vi "Read extParam.vi"(8 "error in":errorcluster, 11 "CRDS Cell Data in":refnum<class "CRDS Cell Data.lvclass">) -> (0 "error out":errorcluster, 2 "extParam":T1={"Tau"=nan, "Tau0cor"=nan, "ext"=nan, "extCorr"=nan, "stdevTau"=nan, "eTau"=nan, "taucorr"=nan, "Tau0"=nan, "max"=nan}, 3 "CRDS Cell Data out":refnum<class "CRDS Cell Data.lvclass">)   [LabVIEW 2018, in "CRDS Lib.lvlib" / "CRDS Cell Data.lvclass"]
uses:
  CRDS Cell Data.lvclass
  Cell/extParam Ctl.ctl
  CRDS Cell Data.lvclass/CRDS Cell Data.ctl
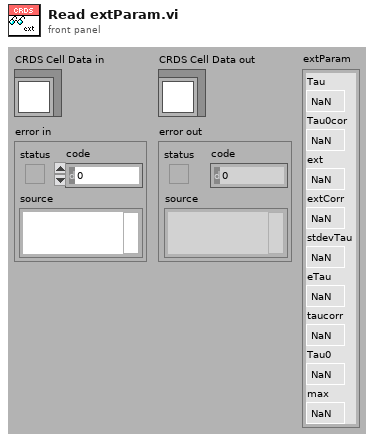
[diagram p1: front panel]
types:
  T1 = typedef "CRDS Lib.lvlib/CRDS Cell Data.lvclass/extParam Ctl.ctl" = cluster{"Tau":sgl, "Tau0cor":sgl, "ext":sgl, "extCorr":sgl, "stdevTau":sgl, "eTau":sgl, "taucorr":sgl, "Tau0":sgl, "max":sgl}
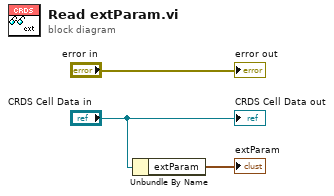
[diagram p0: block diagram]
diagram:
  n1 = Unbundle By Name("CRDS Cell Data in") -> ("extParam"=→"extParam":T1)
  "error out" <- "error in"
  "CRDS Cell Data out" <- "CRDS Cell Data in"
